vi "Read Channels Names.vi"(8 "error in (no error)":errorcluster, 11 "Data List in":refnum<class "Data List.lvclass">) -> (0 "error out":errorcluster, 2 "Channels Names":string[](array[string]), 3 "Data List out":refnum<class "Data List.lvclass">)   [LabVIEW 2020, in "Data List.lvclass"]
uses:
  Data List.lvclass
  Data List.lvclass/Data List.ctl
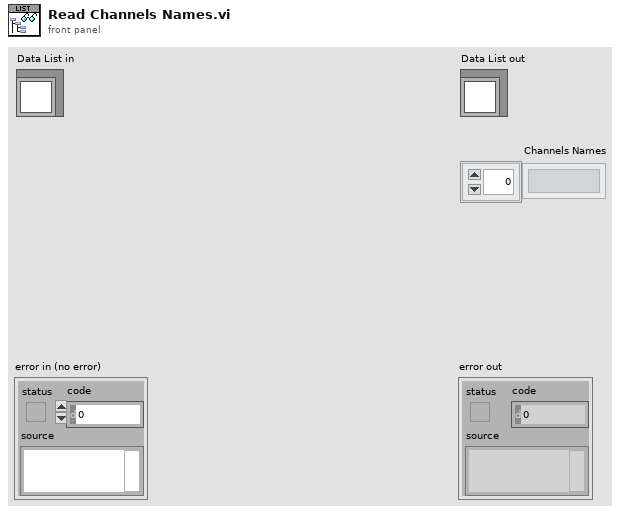
[diagram p1: front panel]
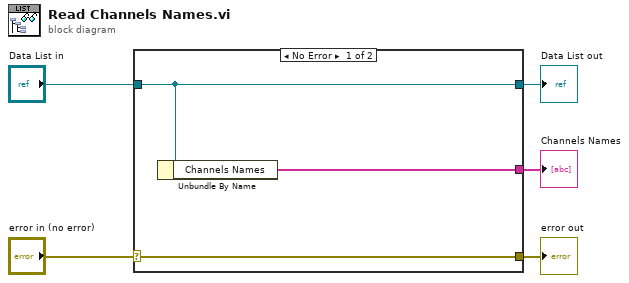
[diagram p0: block diagram]
diagram:
  n1 = case shown="No Error" "error in (no error)" {
    selector: "error in (no error)" -> [w8 w9]
    tunnel: [w8 w9] -> w4
    tunnel: [w7 w10] -> w2
    tunnel: "Data List in" -> [w7 w10]
    tunnel: [w6 _] -> w1
    frame No Error {
      n2 = Unbundle By Name(w7) -> ("Channels Names"=w6:string[])
    }
    frame Error {
    }
  }
  "error out" <- w4
  "Data List out" <- w2
  "Channels Names" <- w1
